vi "Read Input Buffer Size.vi"(8 "error in (no error)":errorcluster, 11 "ONNX Class in":refnum<class "ONNX Class.lvclass">) -> (0 "error out":errorcluster, 2 "Input Buffer Size":i64, 3 "ONNX Class out":refnum<class "ONNX Class.lvclass">)   [LabVIEW 2017, in "ONNX Class Library.lvlib" / "ONNX Class.lvclass"]
uses:
  ONNX Class.lvclass
  ONNX Class.lvclass/ONNX Class.ctl
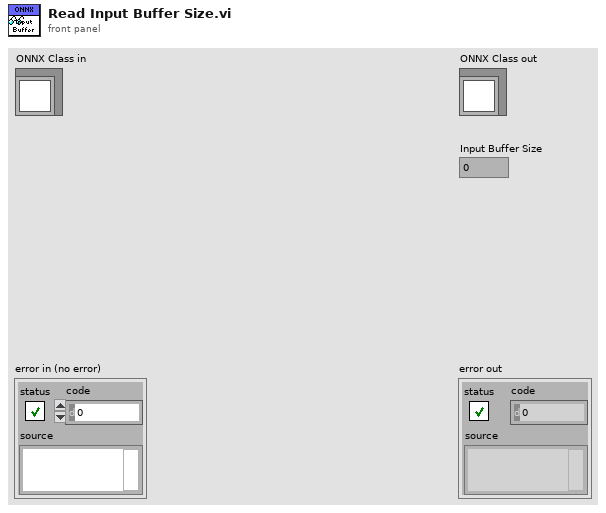
[diagram p1: front panel]
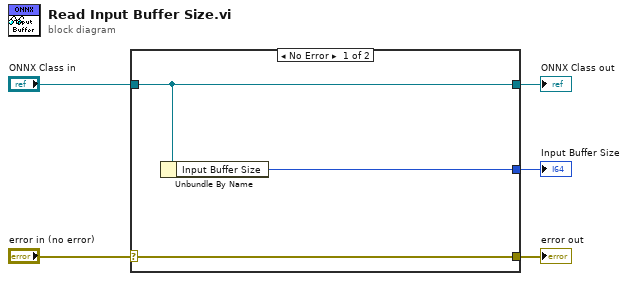
[diagram p0: block diagram]
diagram:
  n1 = case shown="No Error" "error in (no error)" {
    selector: "error in (no error)" -> [w8 w9]
    tunnel: [w8 w9] -> w4
    tunnel: [w7 w10] -> w2
    tunnel: "ONNX Class in" -> [w7 w10]
    tunnel: [w6 _] -> w1
    frame No Error {
      n2 = Unbundle By Name(w7) -> ("Input Buffer Size"=w6:i64)
    }
    frame Error {
    }
  }
  "error out" <- w4
  "ONNX Class out" <- w2
  "Input Buffer Size" <- w1
